vi "Host to DMA one clock test.vi"() -> ()   [LabVIEW 2019]
uses:
  GlobalVars.vi
  <vilib>/FPGAPlugInAG/sbRIO-9606/niLvFpga_Open_sbRIO-9606.vi
  <vilib>/rvi/interface/common/dynamic/niFpgaDynamicAddResources.vi
  <vilib>/FPGAPlugInAG/Dynamic/niLvFpga_Abort_Dynamic.vi
  <vilib>/FPGAPlugInAG/Dynamic/niLvFpga_Reset_Dynamic.vi
  <vilib>/Utility/error.llb/Error Cluster From Error Code.vi
  <vilib>/rvi/errors/niLvFpgaAdjustHostInterfaceError.vi
  <vilib>/FPGAPlugInAG/Dynamic/niLvFpga_Run_Dynamic.vi
  <vilib>/FPGAPlugInAG/Dynamic/niLvFpga_Close_Dynamic.vi
  <vilib>/rvi/interface/nirviOpenFPGA/nirviOpenFPGA.xnode
  FPGA Bitfiles/sbriotest_MainFPGATarget_MainDMAderivedcl_u9ZAtf8s-Ng.lvbitx
  Main DMA derived clock test.vi
  <vilib>/rvi/interface/nirviMethod/nirviMethod.xnode
  <vilib>/rvi/interface/nirviReadWriteControl/nirviReadWriteControl.xnode
  FPGA Bitfiles/sbriotest_SecondFPGATarget_AuxDMAderivedclo_WwoIXhJauaA.lvbitx
  Aux DMA derived clock test.vi
  <vilib>/rvi/interface/nirviCloseFPGA/nirviCloseFPGA.xnode
  NiFpgaLv.dll
  <vilib>/rvi/interface/Simulation/niFpgaSimulationCallBeginRW.vi
  <vilib>/FPGAPlugInAG/Dynamic/niLvFpga_WriteFifo_Dynamic.vi
  <vilib>/rvi/errors/niLvFpgaMergeErrorWithErrorCode.vi
  <vilib>/FPGAPlugInAG/Dynamic/niLvFpga_ReadFifo_Dynamic.vi
panel:
  out "elapsed":u32
  in  "stop":bool
  out "elapsed aux":u32
  out "diff [us]":i32
  out "xt counter":u32
  out "both pass":bool
  out "aux xt counter":u32
  out "xt length":u32
  out "GBIP command":string
  out "xt end":u32
  out "GBIP total":i32
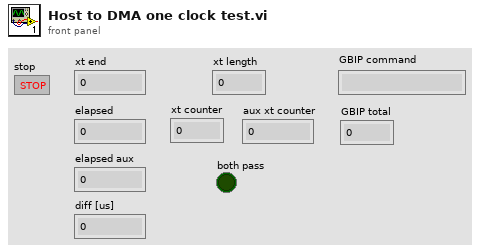
[diagram p1: front panel]
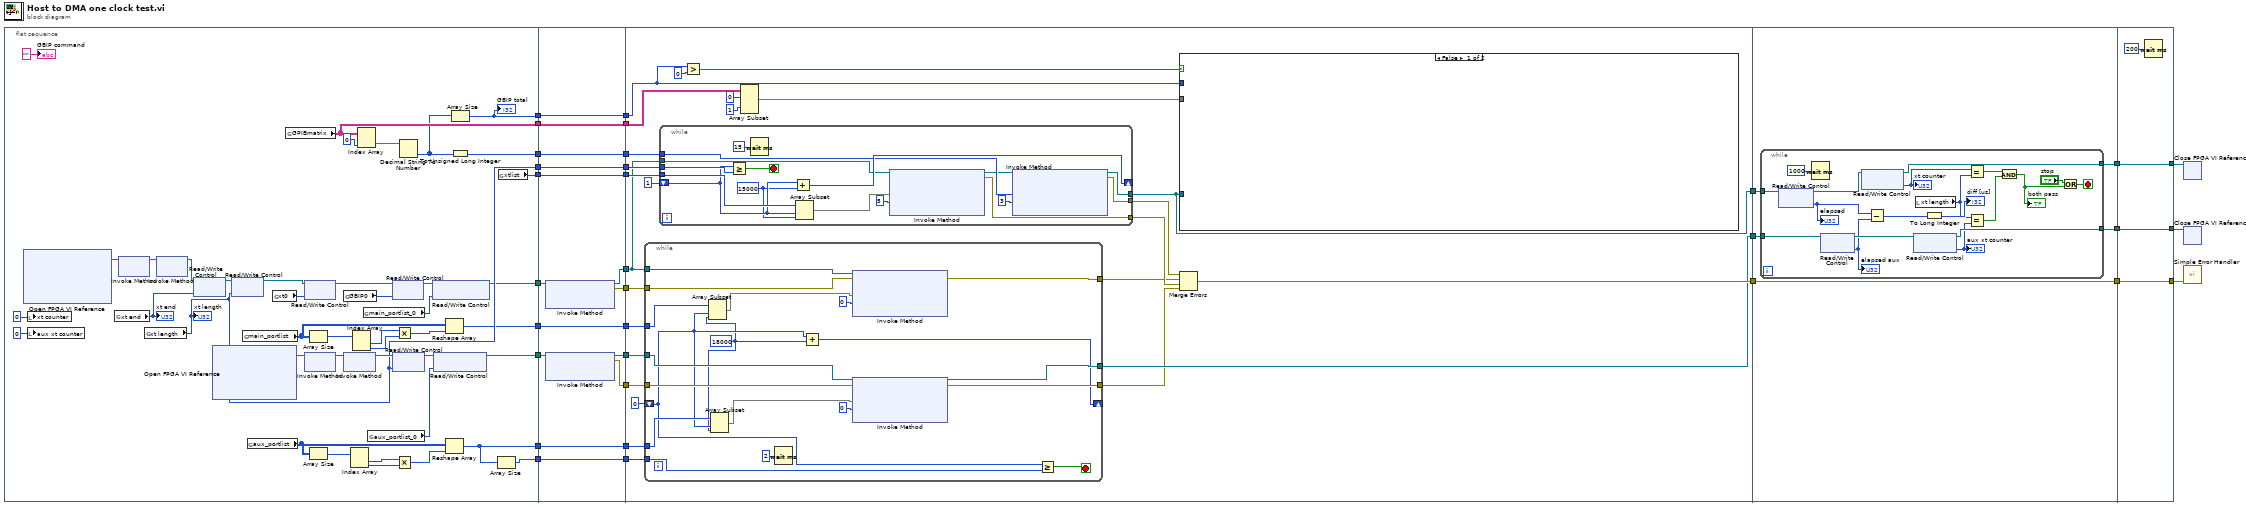
[diagram p0: block diagram]
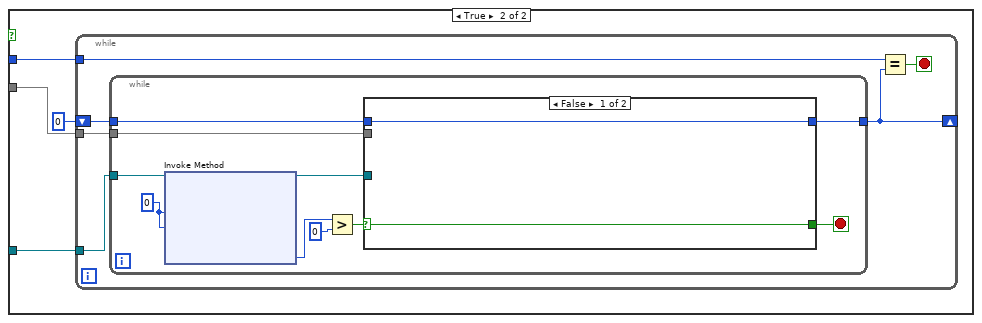
[diagram p2: hidden frame]
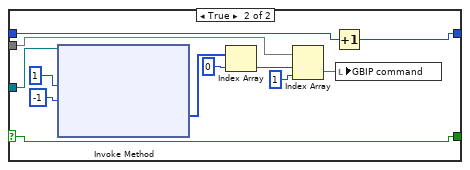
[diagram p3: hidden frame]
diagram:
  n1 = flat-sequence {
    tunnel: [w73] -> w31
    tunnel: [w50] -> w30
    tunnel: [w70] -> w29
    tunnel: [w60] -> w28
    tunnel: [w49] -> w27
    tunnel: [w44] -> w26
    tunnel: [w46] -> w25
    tunnel: [w42] -> w7
    tunnel: [w33] -> w5
    tunnel: [w32] -> w1
    tunnel: w31 -> [w87]
    tunnel: [w87] -> w24
    tunnel: w30 -> [w86]
    tunnel: [w86] -> w23
    tunnel: w29 -> [w85]
    tunnel: [w85] -> w22
    tunnel: w28 -> [w84]
    tunnel: [w84] -> w21
    tunnel: w27 -> [w83]
    tunnel: [w83] -> w20
    tunnel: w26 -> [w82]
    tunnel: w25 -> [w81]
    tunnel: [w80] -> w19
    tunnel: [w79] -> w18
    tunnel: [w78] -> w8
    tunnel: w7 -> [w78]
    tunnel: [w77] -> w6
    tunnel: w5 -> [w77]
    tunnel: [w76] -> w4
    tunnel: [w75] -> w3
    tunnel: [w74] -> w2
    tunnel: w1 -> [w74]
    tunnel: w24 -> [w113]
    tunnel: w23 -> [w111]
    tunnel: w22 -> [w103]
    tunnel: [w96] -> w17
    tunnel: [w108] -> w16
    tunnel: [w107] -> w15
    tunnel: w21 -> [w101]
    tunnel: w20 -> [w106]
    tunnel: w19 -> [w94]
    tunnel: w18 -> [w97]
    tunnel: w8 -> [w93]
    tunnel: w6 -> [w92]
    tunnel: w4 -> [w91]
    tunnel: w3 -> [w90]
    tunnel: w2 -> [w88]
    tunnel: w17 -> [w185]
    tunnel: w16 -> [w184]
    tunnel: w15 -> [w183]
    tunnel: [w187] -> w14
    tunnel: [w186] -> w13
    tunnel: [w184] -> w12
    tunnel: [w208] -> w9
    tunnel: [w209] -> w10
    tunnel: [w210] -> w11
    tunnel: w14 -> [w210]
    tunnel: w13 -> [w209]
    tunnel: w12 -> [w208]
    frame #0 {
      n2 = xnode "Open FPGA VI Reference"() -> ("FPGA VI Reference Out"=w52:refnum<k20>)  [unwired: 2 in, 1 out]
      n3 = local write "xt counter"(u32 0 ("xt counter")) -> ()
      n4 = local write "aux xt counter"(u32 0 ("xt counter")) -> ()
      n5 = global read "GlobalVars.vi" "xt end"() -> (w62:u32)
      "xt end" <- w62
      n6 = xnode "Invoke Method"("FPGA VI Reference In"=w52) -> ("FPGA VI Reference Out"=w63:refnum<k20>)  [unwired: 1 in, 1 out]
      n7 = global read "GlobalVars.vi" "xt length"() -> (w50:u32)
      "xt length" <- w50
      n8 = xnode "Invoke Method"("FPGA VI Reference In"=w63) -> ("FPGA VI Reference Out"=w67:refnum<k20>)  [unwired: 1 in, 1 out]
      n9 = xnode "Read/Write Control"("FPGA VI Reference In"=w67, "xt end"=w62) -> ("FPGA VI Reference Out"=w68:refnum<k20>)  [unwired: 1 in, 1 out]
      n10 = xnode "Open FPGA VI Reference"() -> ("FPGA VI Reference Out"=w51:refnum<k20>)  [unwired: 2 in, 1 out]
      n11 = xnode "Read/Write Control"("FPGA VI Reference In"=w68, "xt total"=w50) -> ("FPGA VI Reference Out"=w59:refnum<k20>)  [unwired: 1 in, 1 out]
      n12 = global read "GlobalVars.vi" "main_portlist"() -> (w48:u16[][])
      n13 = global read "GlobalVars.vi" "aux_portlist"() -> (w37:u16[][])
      n14 = global read "GlobalVars.vi" "xt0"() -> (w54:u32)
      n15 = global read "GlobalVars.vi" "GPIBmatrix"() -> (w70:string[][])
      n16 = xnode "Read/Write Control"("FPGA VI Reference In"=w59, "xt0"=w54) -> ("FPGA VI Reference Out"=w58:refnum<k20>)  [unwired: 1 in, 1 out]
      n17 = xnode "Invoke Method"("FPGA VI Reference In"=w51) -> ("FPGA VI Reference Out"=w64:refnum<k20>)  [unwired: 1 in, 1 out]
      n18 = Array Size(array=w48) -> (size(s)=w47:i32[])
      n19 = Array Size(array=w37) -> (size(s)=w36:i32[])
      n20 = global read "GlobalVars.vi" "GBIP0"() -> (w56:u32)
      n21 = xnode "Invoke Method"("FPGA VI Reference In"=w64) -> ("FPGA VI Reference Out"=w66:refnum<k20>)  [unwired: 1 in, 1 out]
      n22 = Index Array(array=w36) -> (element #1=w35:i32, element #2=w34:i32)  [unwired: 2 in]
      n23 = Index Array(array=w47) -> (element #1=w41:i32, element #2=w40:i32)  [unwired: 2 in]
      n24 = Index Array(array=w70, index (col)=0 ("disabled index (col)")) -> (element=w71:string[])  [unwired: 1 in]
      n25 = global read "GlobalVars.vi" "main_portlist_0"() -> (w43:u16[])
      n26 = global read "GlobalVars.vi" "aux_portlist_0"() -> (w45:u16[])
      n27 = xnode "Read/Write Control"("FPGA VI Reference In"=w66, "xt total"=w50) -> ("FPGA VI Reference Out"=w55:refnum<k20>)  [unwired: 1 in, 1 out]
      n28 = xnode "Read/Write Control"("FPGA VI Reference In"=w58, "GPIB0"=w56) -> ("FPGA VI Reference Out"=w57:refnum<k20>)  [unwired: 1 in, 1 out]
      n29 = Multiply(x=w41, y=w40) -> (x*y=w39:i32)
      n30 = Multiply(x=w35, y=w34) -> (x*y=w38:i32)
      n31 = Decimal String To Number(string=w71) -> (number=w61:i32[])  [unwired: 2 in, 1 out]
      n32 = xnode "Read/Write Control"("FPGA VI Reference In"=w57, "main_portlist_0"=w43) -> ("FPGA VI Reference Out"=w44:refnum<k20>)  [unwired: 1 in, 1 out]
      n33 = xnode "Read/Write Control"("FPGA VI Reference In"=w55, "aux_portlist_0"=w45) -> ("FPGA VI Reference Out"=w46:refnum<k20>)  [unwired: 1 in, 1 out]
      n34 = Reshape Array(w48, w39) -> (w42:u16[])
      n35 = Reshape Array(w37, w38) -> (w33:u16[])
      n36 = To Unsigned Long Integer(number=w61) -> (unsigned 32bit integer=w49:u32[])
      n37 = Array Size(array=w61) -> (size(s)=w60:i32)
      "GBIP total" <- w60
      n38 = Array Size(array=w33) -> (size(s)=w32:i32)
      n39 = global read "GlobalVars.vi" "xtlist"() -> (w73:u32[])
      "GBIP command" <- "" ("GBIP command")
    }
    frame #1 {
      n40 = xnode "Invoke Method"("FPGA VI Reference In"=w82) -> ("FPGA VI Reference Out"=w80:refnum<k20>, "error out"=w76:errorcluster)  [unwired: 2 in]
      n41 = xnode "Invoke Method"("FPGA VI Reference In"=w81) -> ("FPGA VI Reference Out"=w79:refnum<k20>, "error out"=w75:errorcluster)  [unwired: 2 in]
    }
    frame #2 {
      n42 = while {
        tunnel: [w127] -> w98
        tunnel: w97 -> [w132]
        tunnel: [w131] -> w96
        tunnel: [w130] -> w95
        tunnel: w94 -> [w128]
        tunnel: w93 -> [w125]
        tunnel: w92 -> [w124]
        tunnel: w91 -> [w126]
        tunnel: w90 -> [w129]
        shift-right: [w117] -> _
        shift-left: 0 -> [w119]
        tunnel: w88 -> [w120]
        stop <- w121 stop-if-true
        w118 = 18000
        n43 = Array Subset(array=w125, index=w119, length=w118) -> (w123:u16[])
        n44 = Array Subset(array=w124, index=w119, length=w118) -> (w122:u16[])
        n45 = Wait (ms)(milliseconds to wait=u32 2) -> ()  [unwired: 1 out]
        n46 = Add(x=w119, y=w118) -> (x+y=w117:i32)
        n47 = xnode "Invoke Method"("FPGA VI Reference In"=w128, "error in"=w126, "Data"=w123, "Timeout (ms)"=0) -> ("error out"=w127:errorcluster)  [unwired: 2 out]
        n48 = xnode "Invoke Method"("FPGA VI Reference In"=w132, "error in"=w129, "Data"=w122, "Timeout (ms)"=0) -> ("FPGA VI Reference Out"=w131:refnum<k20>, "error out"=w130:errorcluster)  [unwired: 1 out]
        n49 = Greater Or Equal?(x=w119, y=w120) -> (x >= y?=w121:bool)
      }
      n50 = while {
        tunnel: [w182] -> w109
        tunnel: w113 -> [w181]
        shift-right: [w180] -> _
        shift-left: u32 1 -> [w172]
        tunnel: w111 -> [w179]
        tunnel: [w177] -> w110
        tunnel: [w174] -> w107
        tunnel: w106 -> [w173]
        tunnel: w94 -> [w169]
        stop <- w178 stop-if-true
        w171 = u32 15000
        n51 = Greater Or Equal?(x=w172, y=w179) -> (x >= y?=w178:bool)
        n52 = Wait (ms)(milliseconds to wait=u32 15) -> ()  [unwired: 1 out]
        n53 = Add(x=w172, y=w171) -> (x+y=w180:u32)
        n54 = Array Subset(array=w181, index=w172, length=w171) -> (w170:u32[])
        n55 = xnode "Invoke Method"("FPGA VI Reference In"=w169, "Data"=w170, "Timeout (ms)"=5) -> ("FPGA VI Reference Out"=w168:refnum<k20>, "error out"=w182:errorcluster)  [unwired: 1 in, 1 out]
        n56 = xnode "Invoke Method"("FPGA VI Reference In"=w168, "Data"=w173, "Timeout (ms)"=3) -> ("FPGA VI Reference Out"=w174:refnum<k20>, "error out"=w177:errorcluster)  [unwired: 1 in, 1 out]
      }
      n57 = Greater?(x=w101, y=0) -> (0:w99:bool)
      n58 = Array Subset(array=w103, index (row)=0 ("index"), index (col)=1 ("index")) -> (w102:string[][])  [unwired: 2 in]
      n59 = case shown="False" w99 {
        tunnel: w107 -> [_ w136]
        tunnel: w102 -> [_ w135]
        tunnel: w101 -> [_ w134]
        frame False {
        }
        frame True {
          n60 = while {
            tunnel: w136 -> [w142]
            tunnel: w135 -> [w141]
            shift-right: [w138] -> _
            shift-left: 0 -> [w140]
            tunnel: w134 -> [w137]
            stop <- w139 stop-if-true
            n61 = while {
              tunnel: w142 -> [w152]
              tunnel: w141 -> [w151]
              tunnel: w140 -> [w146]
              tunnel: [w145] -> w138
              stop <- w144 stop-if-true
              w143 = u32 0 ("Timeout (ms)")
              n62 = xnode "Invoke Method"("FPGA VI Reference In"=w152, "Number of Elements"=w143, "Timeout (ms)"=w143) -> ("FPGA VI Reference Out"=w150:refnum<k20>, "Elements Remaining"=w148:u32)  [unwired: 1 in, 2 out]
              n63 = Greater?(x=w148, y=u32 0) -> (0:w147:bool)
              n64 = case shown="False" w147 {
                selector: w147 -> [w153 w155]
                tunnel: w151 -> [_ w166]
                tunnel: w150 -> [_ w165]
                tunnel: w146 -> [w154 w157]
                tunnel: [w154 w156] -> w145
                tunnel: [w153 w155] -> w144
                frame False {
                }
                frame True {
                  n65 = xnode "Invoke Method"("FPGA VI Reference In"=w165, "Number of Elements"=u32 1, "Timeout (ms)"=-1) -> ("Data"=w162:u16[])  [unwired: 1 in, 3 out]
                  n66 = Index Array(array=w162, index=0) -> (element=w160:u16)
                  n67 = Index Array(array=w166, index (row)=w160, index (col)=1 ("disabled index (col)")) -> (element=w158:string)
                  n68 = Increment(x=w157) -> (x+1=w156:i32)
                  n69 = local write "GBIP command"(w158) -> ()
                }
              }
            }
            n70 = Equal?(x=w137, y=w138) -> (x = y?=w139:bool)
          }
        }
      }
      n71 = Merge Errors(w110, w98, w109, w95) -> (w108:errorcluster)
    }
    frame #3 {
      n72 = while {
        tunnel: [w196] -> w187
        tunnel: [w200] -> w186
        tunnel: w185 -> [w199]
        tunnel: w183 -> [w197]
        stop <- w194 stop-if-true
        n73 = xnode "Read/Write Control"("FPGA VI Reference In"=w197) -> ("FPGA VI Reference Out"=w201:refnum<k20>, "elapsed"=w198:u32)  [unwired: 1 in, 1 out]
        "elapsed" <- w198
        n74 = Wait (ms)(milliseconds to wait=u32 1000) -> ()  [unwired: 1 out]
        n75 = xnode "Read/Write Control"("FPGA VI Reference In"=w199) -> ("FPGA VI Reference Out"=w206:refnum<k20>, "elapsed"=w205:u32)  [unwired: 1 in, 1 out]
        "elapsed aux" <- w205
        n76 = xnode "Read/Write Control"("FPGA VI Reference In"=w201) -> ("FPGA VI Reference Out"=w200:refnum<k20>, "xt counter"=w192:u32)  [unwired: 1 in, 1 out]
        "xt counter" <- w192
        n77 = Subtract(x=w198, y=w205) -> (x-y=w204:u32)
        n78 = xnode "Read/Write Control"("FPGA VI Reference In"=w206) -> ("FPGA VI Reference Out"=w196:refnum<k20>, "xt counter"=w193:u32)  [unwired: 1 in, 1 out]
        "aux xt counter" <- w193
        n79 = local read "xt length"() -> (w191:u32)
        n80 = To Long Integer(number=w204) -> (32bit integer=→"diff [us]":i32)
        n81 = Equal?(x=w192, y=w191) -> (x = y?=w190:bool)
        n82 = Equal?(x=w191, y=w193) -> (x = y?=w189:bool)
        n83 = And(x=w190, y=w189) -> (x .and. y?=w188:bool)
        "both pass" <- w188
        n84 = Or(x="stop", y=w188) -> (x .or. y?=w194:bool)
      }
    }
    frame #4 {
      n85 = Wait (ms)(milliseconds to wait=u32 200) -> ()  [unwired: 1 out]
    }
  }
  n86 = xnode "Close FPGA VI Reference"("FPGA VI Reference In"=w10) -> ()  [unwired: 1 in, 1 out]
  n87 = xnode "Close FPGA VI Reference"("FPGA VI Reference In"=w11) -> ()  [unwired: 1 in, 1 out]
  n88 = call <vilib>:"Simple Error Handler.vi"("error in (no error)"=w9) -> ()  [unwired: 4 in, 5 out]
